vi "destroy.vi"(8 "error in (no error)":errorcluster, 11 "TaskController in":refnum<class "TaskController.lvclass">) -> (0 "error out":errorcluster, 2 "taskError":errorcluster, 3 "taskResult":refnum<class "ITask.lvclass">)   [LabVIEW 2023, in "TLC_Daemon.lvlib" / "TaskController.lvclass"]
doc: "Destroys the TaskController and returns the task outputs: Task out and Error out.\n\nIf the task is running, this method forces it to stop. If the Destroy method is called before the task has been launched, or if the task fails to stop, the Task object originally provided to the New method is returned.\n\nSet 'destroyStopMechanism' to True to also trigger the destruction of the StopMechanism.\n_____________________________________\nTLC Daemon 1.0.0.2\nCopyright (c) 2026 Andrea Cadei"
uses:
  TaskController.lvclass
  ITask/ITask.lvclass
  TaskController.lvclass/TaskController.ctl
  ITaskStopMechanism/ITaskStopMechanism.lvclass
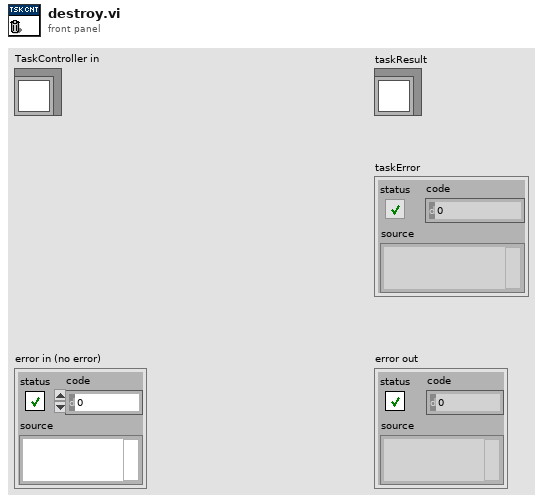
[diagram p1: front panel]
types:
  T1 = typedef "TLC_Daemon.lvlib/TaskController.lvclass/status.ctl" = enum16{"NotReady", "Ready", "Running", "Stopped", "Unknown"}
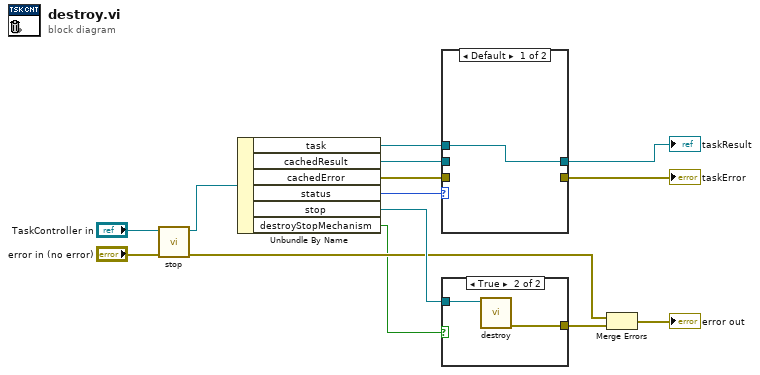
[diagram p0: block diagram]
diagram:
  n1 = call "stop.vi"("error in (no error)"="error in (no error)", "TaskController in"="TaskController in") -> ("error out"=w8:errorcluster, "TaskController out"=w13:refnum<class "TaskController.lvclass">)  [unwired: 8 in]
  n2 = Unbundle By Name(w13) -> ("task"=w2:refnum<class "ITask.lvclass">, "cachedResult"=w6:refnum<class "ITask.lvclass">, "cachedError"=w4:errorcluster, "status"=w7:T1, "stop"=w12:refnum<class "ITaskStopMechanism.lvclass">, "destroyStopMechanism"=w1:bool)
  n3 = case shown="Default" w7 {
    tunnel: w6 -> [_ w17]
    tunnel: [w15 w17] -> w5
    tunnel: w4 -> [_ w16]
    tunnel: [_ w16] -> w3
    tunnel: w2 -> [w15 _]
    frame Default {
    }
    frame "Stopped" {
      # "If task has stopped properly, returns cached result and error"
    }
  }
  "taskResult" <- w5
  "taskError" <- w3
  n4 = case shown="True" w1 {
    tunnel: w12 -> [_ w19]
    tunnel: [_ w18] -> w11
    frame False {
    }
    frame True {
      n5 = call-dynamic "destroy.vi"("ITaskStopMechanism in"=w19) -> ("error out"=w18:errorcluster)  [unwired: 9 in, 1 out]
    }
  }
  n6 = Merge Errors(w8, w11) -> (→"error out":errorcluster)
